vi "Control_Event.vi"(8 "error in":errorcluster, 10 "Estado":T1) -> (0 "error out":errorcluster, 2 "user event out":refnum<user-event>)   [LabVIEW 2026]
uses:
  Control/Ctrl_GuiEvent.ctl
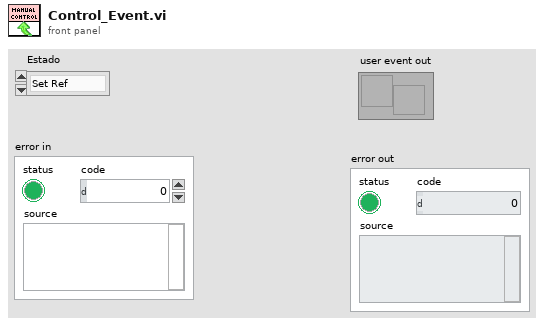
[diagram p1: front panel]
types:
  T1 = typedef "Ctrl_GuiEvent.ctl" = enum16{"Set Ref", "Update Enc", "Stop", "Get Ref"}
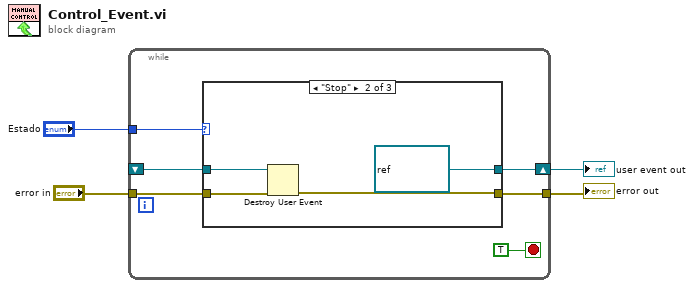
[diagram p0: block diagram]
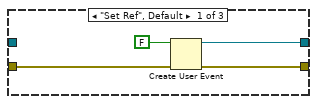
[diagram p2: hidden frame]
diagram:
  n1 = while {
    tunnel: "error in" -> [w9]
    tunnel: "Estado" -> [w10]
    tunnel: [w8] -> w2
    shift-right: [w6] -> w1
    shift-left: _ -> [w5]
    stop <- TRUE stop-if-true
    n2 = case shown="\"Stop\"" w10 {
      tunnel: w9 -> [w13 w18 w20]
      tunnel: [w12 w17 w20] -> w8
      tunnel: [w11 refnum<user-event> refnum ("user event out") w19] -> w6
      tunnel: w5 -> [_ w15 w19]
      frame "Set Ref", Default {
        n3 = Create User Event(user event datatype=FALSE ("booles"), error in=w13) -> (user event=w11:refnum<user-event>, error out=w12:errorcluster)
      }
      frame "Stop" {
        n4 = Destroy User Event(user event=w15, error in=w18) -> (error out=w17:errorcluster)
      }
      frame "Get Ref" {
      }
    }
  }
  "error out" <- w2
  "user event out" <- w1
